vi "mainObjectivesRegistrationNew.vi"() -> ()   [LabVIEW 2017]
uses:
  globalDevices.vi
  globalUtilities.vi
panel:
  in  "galvo DY (V)":dbl=0.155
  in  "galvo DX (V)":dbl=0.145
  out "N^2 +M galvo":i32
  out "curr. piezo pos (index)":i32
  out "curr. galvo pos (index)":i32
  out "opendisplayvolume":bool=TRUE
  out "set piezo pos (um)":dbl
  in  "frames per second":dbl=5.0
  in  "piezo2 M-1":i32=20
  in  "galvo N-1":i32=3
  # "REGISTRATION BETWEEN GALVO AND CAMERA"
  # "Acquisition parameters"
  # "# of piezo positions to scan"
  # "sqrt# of galvo positions in grid\n(without symmetry breaking)"
  # "1. After the piezo scan ends, open the Display Volume vi to select a rectangle to locate the\n    two-photon spot.\n2. After the galvo scan ends, open the vi again and select a point where you want to shine\n    light, to test the registration."
  # "When this button is on, open the VI\nsubvi/subvi-acquisitionUtilities/acquisitionDisplayVolume.vi"
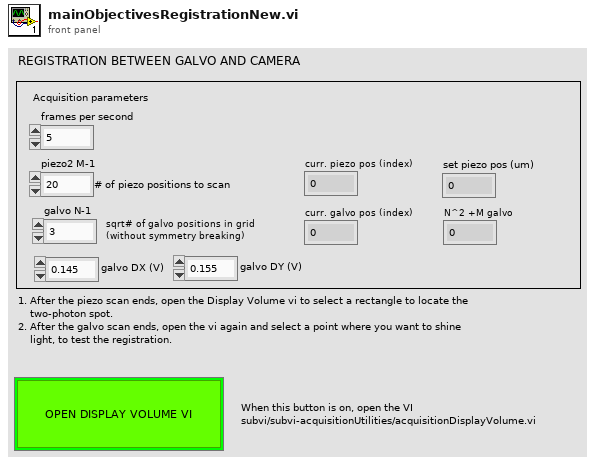
[diagram p1: front panel]
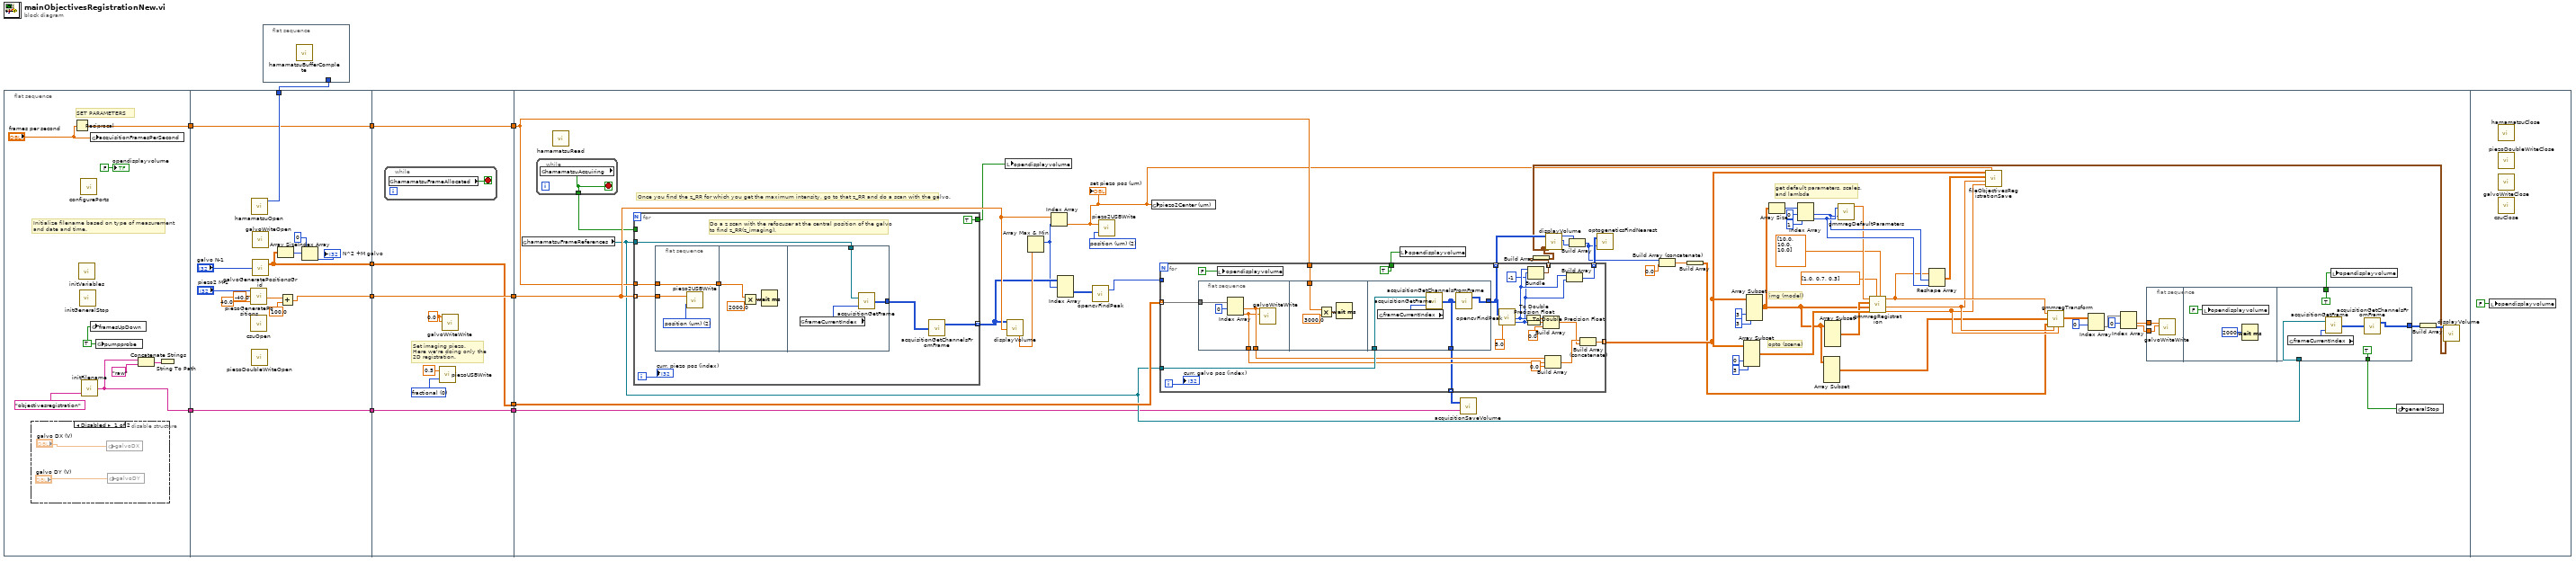
[diagram p0: block diagram]
diagram:
  n1 = flat-sequence {
    tunnel: [w15] -> w8
    tunnel: [w12] -> w1
    tunnel: [w34] -> w11
    tunnel: [w27] -> w10
    tunnel: w8 -> [w30]
    tunnel: [w30] -> w6
    tunnel: [w26] -> w4
    tunnel: [w22] -> w2
    tunnel: w1 -> [w22]
    tunnel: w10 -> [w40]
    tunnel: [w40] -> w9
    tunnel: [w39] -> w7
    tunnel: w6 -> [w39]
    tunnel: [w38] -> w5
    tunnel: w4 -> [w38]
    tunnel: [w36] -> w3
    tunnel: w2 -> [w36]
    tunnel: w9 -> [w99]
    tunnel: w7 -> [w90]
    tunnel: w5 -> [w93]
    tunnel: w3 -> [w44]
    frame #0 {
      w13 = TRUE ("pumpprobe")
      # "SET PARAMETERS"
      # "Initialize filename based on type of measurement\nand date and time."
      n2 = disable-structure shown="Disabled" {
        frame Disabled {
          n3 = global write "globalDevices.vi" "galvoDX"("galvo DX (V)") -> ()
          n4 = global write "globalDevices.vi" "galvoDY"("galvo DY (V)") -> ()
        }
        frame Enabled {
        }
      }
      n5 = Reciprocal(x="frames per second") -> (1/x=w15:dbl)
      n6 = call "initVariables.vi"() -> ()  [unwired: 12 in]
      n7 = call "initGeneralStop.vi"() -> ()  [unwired: 1 in]
      n8 = call "configurePorts.vi"() -> ()  [unwired: 12 in]
      n9 = call "initFilename.vi"("Experiment type"="objectivesregistration") -> ("folder name"=w12:string)  [unwired: 1 in]
      n10 = global write "globalUtilities.vi" "framesUpDown"(w13) -> ()
      n11 = global write "globalUtilities.vi" "acquisitionFramesPerSecond"("frames per second") -> ()
      n12 = global write "globalUtilities.vi" "pumpprobe"(w13) -> ()
      n13 = Concatenate Strings(w12, "raw") -> (w19:string)
      n14 = String To Path(string=w19) -> ()  [unwired: 1 out]
      "opendisplayvolume" <- FALSE ("OPEN DISPLAY VOLUME")
    }
    frame #1 {
      n15 = call "piezoGeneratePositions.vi"("zf"=40.0, "z0"=-40.0, "M"="piezo2 M-1") -> ("positions (z)"=w29:dbl[])
      n16 = call "csuOpen.vi"() -> ()  [unwired: 14 in, 2 out]
      n17 = call "hamamatsuOpen.vi"() -> ("Handle out"=w34:u32)  [unwired: 3 out]
      n18 = call "piezoDoubleWriteOpen.vi"() -> ()  [unwired: 2 in]
      n19 = call "galvoWriteOpen.vi"() -> ()  [unwired: 12 in]
      n20 = call "galvoGeneratePositionsGrid.vi"("N-1"="galvo N-1") -> ("grid"=w26:dbl[][])  [unwired: 1 out]
      n21 = Array Size(array=w26) -> (size(s)=w25:i32[])
      n22 = Add(x=w29, y=100.0) -> (x+y=w27:dbl[])
      n23 = Index Array(array=w25, index=0) -> (element=→"N^2 +M galvo":i32)
    }
    frame #2 {
      w37 = 0.0 ("X")
      w42 = u16 0 items=["fractional", "voltage (V)", "position (um)"] ("mode")
      # "Set imaging piezo.\nHere we're doing only the\n2D registration."
      n24 = while {
        stop <- w43 stop-if-true
        n25 = global read "globalDevices.vi" "hamamatsuFrameAllocated"() -> (w43:bool)
      }
      n26 = call "piezoUSBWrite.vi"("mode"=w42, "position"=0.5) -> ()  [unwired: 1 in]
      n27 = call "galvoWriteWrite.vi"("X"=w37, "Y"=w37) -> ()  [unwired: 4 in]
    }
    frame #3 {
      w98 = u16 2 items=["fractional", "voltage (V)", "position (um)"] ("mode")
      # "get default parameters, scales,\nand lambda"
      # "img (model)"
      # "opto (scene)"
      # "Once you find the z_RR for which you get the maximum intensity, go to that z_RR and do a scan with the galvo."
      n28 = global read "globalDevices.vi" "hamamatsuFrameReferences"() -> (w69:refnum<data-value>[])
      n29 = while {
        tunnel: [w162] -> w92
        stop <- w162 stop-if-true
        n30 = global read "globalUtilities.vi" "hamamatsuAcquiring"() -> (w162:bool)
      }
      n31 = call "hamamatsuRead.vi"() -> ()  [unwired: 12 in]
      n32 = for {
        tunnel: w69 -> [w151]
        tunnel: w99 -> [w152] mode=indexing
        tunnel: w90 -> [w150]
        tunnel: [TRUE] -> w94
        tunnel: [w145] -> w97 mode=indexing
        tunnel: w92 -> [_]
        i -> [w147]
        # "Do a z scan with the refocuser at the central position of the galvo \nto find z_RR(z_imaging)."
        n33 = flat-sequence {
          tunnel: w152 -> [w155]
          tunnel: w150 -> [w153]
          tunnel: [w153] -> w149
          tunnel: w149 -> [w156]
          tunnel: w151 -> [w160]
          tunnel: [w159] -> w146
          frame #0 {
            w154 = u16 2 items=["fractional", "voltage (V)", "position (um)"] ("mode")
            n34 = call "piezo2USBWrite.vi"("mode"=w154, "position"=w155) -> ()  [unwired: 1 in]
          }
          frame #1 {
            n35 = Multiply(x=w156, y=2000.0) -> (x*y=w158:dbl)
            n36 = Wait (ms)(milliseconds to wait=w158) -> ()  [unwired: 1 out]
          }
          frame #2 {
            n37 = global read "globalUtilities.vi" "frameCurrentIndex"() -> (w161:i32)
            n38 = call "acquisitionGetFrame.vi"("index"=w161, "hamamatsuFrameReferences"=w160) -> ("frameOut"=w159:u16[][])
          }
        }
        n39 = call "acquisitionGetChannelsFromFrame.vi"("frameIn"=w146) -> ("Red"=w145:u16[][])  [unwired: 1 out]
        "curr. piezo pos (index)" <- w147
      }
      n40 = local write "opendisplayvolume"(w94) -> ()
      n41 = call "displayVolume.vi"("frames"=w97, "z"=w99) -> ("z profile"=w100:dbl[])  [unwired: 12 in, 5 out]
      n42 = Array Max & Min(array=w100) -> (max index (indices)=w96:i32)  [unwired: 3 out]
      n43 = Index Array(array=w99, index=w96) -> (element=w46:dbl)
      "set piezo pos (um)" <- w46
      n44 = Index Array(array=w97, index (dim 0)=w96) -> (element=w95:u16[][])  [unwired: 2 in]
      n45 = call "opencvFindPeak.vi"("Image (2D)"=w95) -> ("maxLocX"=w91:i32)  [unwired: 1 in, 1 out]
      n46 = call "piezo2USBWrite.vi"("mode"=w98, "position"=w46) -> ()  [unwired: 1 in]
      n47 = global write "globalDevices.vi" "piezo2Center (um)"(w46) -> ()
      n48 = for {
        tunnel: w93 -> [w133] mode=indexing
        tunnel: w91 -> [_]
        tunnel: w90 -> [w132]
        tunnel: w69 -> [w131]
        tunnel: [w128] -> w89 mode=indexing
        tunnel: [w127] -> w48 mode=indexing
        tunnel: [w119] -> w75 mode=indexing
        tunnel: [w117] -> w72 mode=indexing
        tunnel: [TRUE ("OPEN DISPLAY VOLUME")] -> w50
        tunnel: [w111] -> w45 mode=indexing
        i -> [w129]
        n49 = flat-sequence {
          tunnel: w133 -> [w137]
          tunnel: [w135] -> w123
          tunnel: [w134] -> w122
          tunnel: w132 -> [w139]
          tunnel: w131 -> [w143]
          tunnel: [w142] -> w128
          tunnel: [w141] -> w111
          frame #0 {
            n50 = Index Array(array=w137, index #1=0 ("index")) -> (element #1=w135:dbl, element #2=w134:dbl)  [unwired: 1 in]
            n51 = call "galvoWriteWrite.vi"("X"=w135, "Y"=w134) -> ()  [unwired: 4 in]
          }
          frame #1 {
            n52 = Multiply(x=w139, y=3000.0) -> (x*y=w138:dbl)
            n53 = Wait (ms)(milliseconds to wait=w138) -> ()  [unwired: 1 out]
          }
          frame #2 {
            n54 = global read "globalUtilities.vi" "frameCurrentIndex"() -> (w144:i32)
            n55 = call "acquisitionGetFrame.vi"("index"=w144, "hamamatsuFrameReferences"=w143) -> ("frameOut"=w141:u16[][])
            n56 = call "acquisitionGetChannelsFromFrame.vi"("frameIn"=w141) -> ("Red"=w142:u16[][])  [unwired: 1 out]
          }
        }
        n57 = local write "opendisplayvolume"(FALSE ("OPEN DISPLAY VOLUME")) -> ()
        n58 = call "opencvFindPeak.vi"("blur"=5.0, "Image (2D)"=w128) -> ("maxLocY"=w116:i32, "maxLocX"=w118:i32)
        n59 = To Double Precision Float(number=w118) -> (double precision float=w125:dbl)
        n60 = To Double Precision Float(number=w116) -> (double precision float=w124:dbl)
        n61 = Bundle("maxLocX"=w118, "maxLocY"=w116, -1) -> (w127:cluster{"maxLocX":i32, "maxLocY":i32, i32})  [unwired: 1 in]
        n62 = Build Array(w125, w124, 0.0 ("element")) -> (w115:dbl[])
        n63 = Build Array(w123, w122, 0.0 ("element")) -> (w120:dbl[])
        n64 = Build Array(w118, w116) -> (w117:i32[])
        n65 = Build Array (concatenate)(w120, w115) -> (w119:dbl[])
        "curr. galvo pos (index)" <- w129
      }
      n66 = local write "opendisplayvolume"(w50) -> ()
      n67 = call "acquisitionSaveVolume.vi"("folder"=w44, "volume"=w45) -> ()  [unwired: 1 in]
      n68 = Build Array(w48) -> (w47:cluster{"maxLocX":i32, "maxLocY":i32, i32}[][])
      n69 = call "displayVolume.vi"("frames"=w89, "overlay (z:-1 all planes)"=w47) -> ("X0out"=w88:i32, "Y0out"=w87:i32)  [unwired: 12 in, 4 out]
      n70 = Build Array(w88, w87) -> (w54:i32[])
      n71 = call "optogeneticsFindNearest.vi"("point"=w54, "points"=w72) -> ()  [unwired: 1 out]
      n72 = Build Array (concatenate)(w54, 0.0) -> (w52:dbl[])
      n73 = Build Array(w52) -> (w51:dbl[][])
      n74 = Array Subset(array=w75, index (col)=0 ("index"), length (col)=3 ("length")) -> (w64:dbl[][])  [unwired: 2 in]
      n75 = Array Subset(array=w75, index (col)=3 ("index"), length (col)=3 ("length")) -> (w62:dbl[][])  [unwired: 2 in]
      n76 = Array Size(array=w62) -> (size(s)=w82:i32[])
      n77 = Index Array(array=w82, index #1=0 ("index"), index #2=1 ("index")) -> (element #1=w84:i32, element #2=w85:i32)
      n78 = Array Subset(array=w62) -> (w61:dbl[][])  [unwired: 4 in]
      n79 = Array Subset(array=w62) -> (w63:dbl[][])  [unwired: 4 in]
      n80 = call "gmmregDefaultParameters.vi"("D (3)"=w85, "nctrlPts"=w84) -> ("param0"=w83:dbl[])  [unwired: 3 out]
      n81 = call "gmmregRegistration.vi"("lambda"=dbl[] [10.0, 10.0, 10.0], "scale"=dbl[] [1.0, 0.7, 0.3], "scene"=w64, "model"=w62, "ctrlPoints"=w63, "param0"=w83) -> ("denormParams out"=w65:dbl[], "normParams out"=w73:dbl[], "param0 out"=w74:dbl[])  [unwired: 2 in, 1 out]
      n82 = Reshape Array(w74, w84, w85) -> (w86:dbl[][])
      n83 = call "fileObjectivesRegistrationSave.vi"("xyz(opto)xyz(img)"=w75, "param"=w86, "normParam"=w73, "denormParam"=w65, "z(opto)z(img)"=w46) -> ()  [unwired: 1 in]
      n84 = call "gmmregTransform.vi"("param0"=w74, "ctrlPts"=w61, "pts"=w51, "normParams"=w73, "denormParams"=w65) -> ("out"=w71:dbl[][])  [unwired: 4 in]
      n85 = Index Array(array=w71, index (row)=0) -> (element=w60:dbl[])  [unwired: 1 in]
      n86 = Index Array(array=w60, index #1=0 ("index")) -> (element #1=w58:dbl, element #2=w57:dbl)  [unwired: 1 in]
      n87 = flat-sequence {
        tunnel: w58 -> [w102]
        tunnel: w57 -> [w101]
        tunnel: w69 -> [w109]
        tunnel: [w105] -> w68
        tunnel: [TRUE] -> w66
        tunnel: [TRUE ("opendisplayvolume")] -> w49
        frame #0 {
          n88 = call "galvoWriteWrite.vi"("X"=w102, "Y"=w101) -> ()  [unwired: 4 in]
        }
        frame #1 {
          n89 = local write "opendisplayvolume"(FALSE ("opendisplayvolume")) -> ()
          n90 = Wait (ms)(milliseconds to wait=u32 2000) -> ()  [unwired: 1 out]
        }
        frame #2 {
          n91 = global read "globalUtilities.vi" "frameCurrentIndex"() -> (w110:i32)
          n92 = call "acquisitionGetFrame.vi"("index"=w110, "hamamatsuFrameReferences"=w109) -> ("frameOut"=w106:u16[][])
          n93 = call "acquisitionGetChannelsFromFrame.vi"("frameIn"=w106) -> ("Red"=w105:u16[][])  [unwired: 1 out]
        }
      }
      n94 = local write "opendisplayvolume"(w49) -> ()
      n95 = global write "globalUtilities.vi" "generalStop"(w66) -> ()
      n96 = Build Array(w68) -> (w67:u16[][][])
      n97 = call "displayVolume.vi"("frames"=w67, "overlay (z:-1 all planes)"=w47) -> ()  [unwired: 12 in, 6 out]
    }
    frame #4 {
      n98 = local write "opendisplayvolume"(FALSE ("opendisplayvolume")) -> ()
      n99 = call "hamamatsuClose.vi"() -> ()  [unwired: 1 out]
      n100 = call "piezoDoubleWriteClose.vi"() -> ()  [unwired: 1 in]
      n101 = call "galvoWriteClose.vi"() -> ()  [unwired: 12 in]
      n102 = call "csuClose.vi"() -> ()  [unwired: 12 in]
    }
  }
  n103 = flat-sequence {
    tunnel: w11 -> [_]
    frame #0 {
      n104 = call "hamamatsuBufferComplete.vi"() -> ()  [unwired: 12 in]
    }
  }
